vi "SoulEatingEnchantment_Create.vi"(8 "Error In":errorcluster, 11 "reference in":refnum<class "SoulEatingEnchantment.lvclass">) -> (0 "Error Out":errorcluster, 3 "reference out":refnum<class "SoulEatingEnchantment.lvclass">)   [LabVIEW 2020, in "SoulEatingEnchantment.lvclass"]
uses:
  SoulEatingEnchantment.lvclass
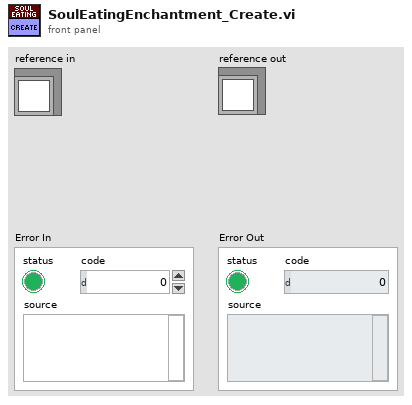
[diagram p1: front panel]
types:
  T1 = typedef "SoulEatingEnchantment.lvclass/ObjectAttributes.ctl" = cluster{"None":bool}
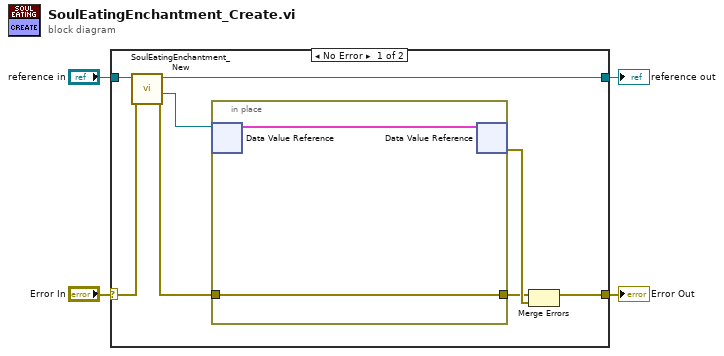
[diagram p0: block diagram]
diagram:
  n1 = case shown="No Error" "Error In" {
    selector: "Error In" -> [w11 w16]
    tunnel: [w5 w16] -> w3
    tunnel: "reference in" -> [w12 w15]
    tunnel: [w10 w15] -> w1
    frame No Error {
      n2 = call "SoulEatingEnchantment_New.vi"("error in (no error)"=w11, "reference in"=w12) -> ("error out"=w7:errorcluster, "DVRRefOut"=w8:refnum<data-value>, "reference out"=w10:refnum<class "SoulEatingEnchantment.lvclass">)  [unwired: 6 in, 1 out]
      n3 = in-place {
        in-place-border: w7 -> [w14]
        in-place-border: [w14] -> w6
        n4 = in-place-dvr #1(w8) -> (w13:T1)  [unwired: 1 out]
        n5 = in-place-dvr #1(w13) -> (w9:errorcluster)  [unwired: 1 out]
      }
      n6 = Merge Errors(w6, w9) -> (w5:errorcluster)
    }
    frame Error {
      # "VI-TechBaseTemplate_Simple_4x4x4"
    }
  }
  "Error Out" <- w3
  "reference out" <- w1
